vi "readRegister4.vi"() -> ()   [LabVIEW 2009]
panel:
  in  "Port":u16=9764
  in  "IP":string="172.16.7.43"
  out "Register value":u32
  in  "Device":u16(ring)=4 items=["Attenuation", "Clipping", "Enable channel", "Delay line", "ASIC"]
  out "error out":errorcluster
  in  "error in":errorcluster
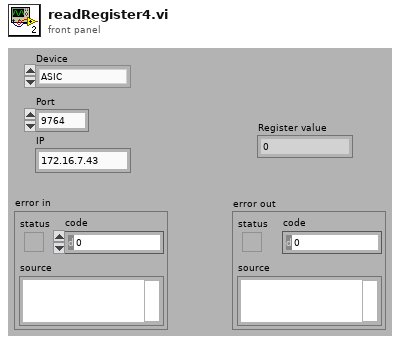
[diagram p1: front panel]
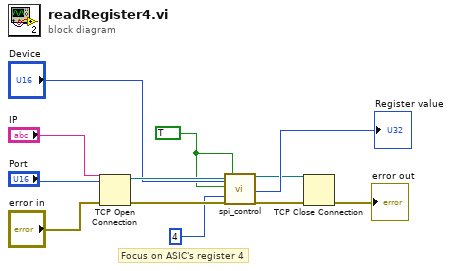
[diagram p0: block diagram]
diagram:
  w4 = TRUE
  # "Focus on ASIC's register 4"
  n1 = TCP Open Connection(address="IP", remote port or service name="Port", error in (no error)="error in") -> (connection ID=w9:refnum<k5>, error out=w10:errorcluster)  [unwired: 2 in]
  n2 = call "spi_control.vi"("connection ID"=w9, "Device"="Device", "Read/#write"=w4, "Register or channel"=4, "error out 3"=w10, "Read physical"=w4) -> ("connection ID out"=w2:refnum<k5>, "data read value"=→"Register value":u32, "error out 2"=w1:errorcluster)  [unwired: 6 in, 5 out]
  n3 = TCP Close Connection(connection ID=w2, error in (no error)=w1) -> (error out=→"error out":errorcluster)  [unwired: 1 in, 1 out]
